vi "Parse string.vi"(11 "Address":string) -> (0 "Len":u8, 1 "StartAddress":u32, 2 "DataBlock":u16, 3 "Memory Area":T1=enum."DB Area")   [LabVIEW 2025, in "SIMATIC_S7.lvclass"]
uses:
  SIMATIC_S7.lvclass
  <vilib>/Hampel Software Engineering/S7NetCom/Source/Controls/S7_Memory_Area.ctl
  <vilib>/regexp/Match Regular Expression.xnode
  <vilib>/Hampel Software Engineering/S7NetCom/Source/S7NetCom.lvclass
panel:
  # "DB6010.40[28]"
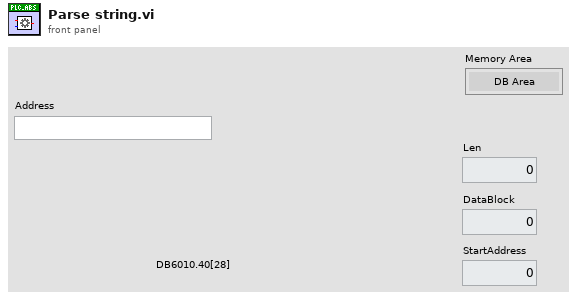
[diagram p1: front panel]
types:
  T1 = typedef "S7NetCom.lvlib/S7NetCom.lvclass/S7_Memory_Area.ctl" = enum8{"P Area", "I Area", "O Area", "M Area", "DB Area", "Counter", "Timer"}
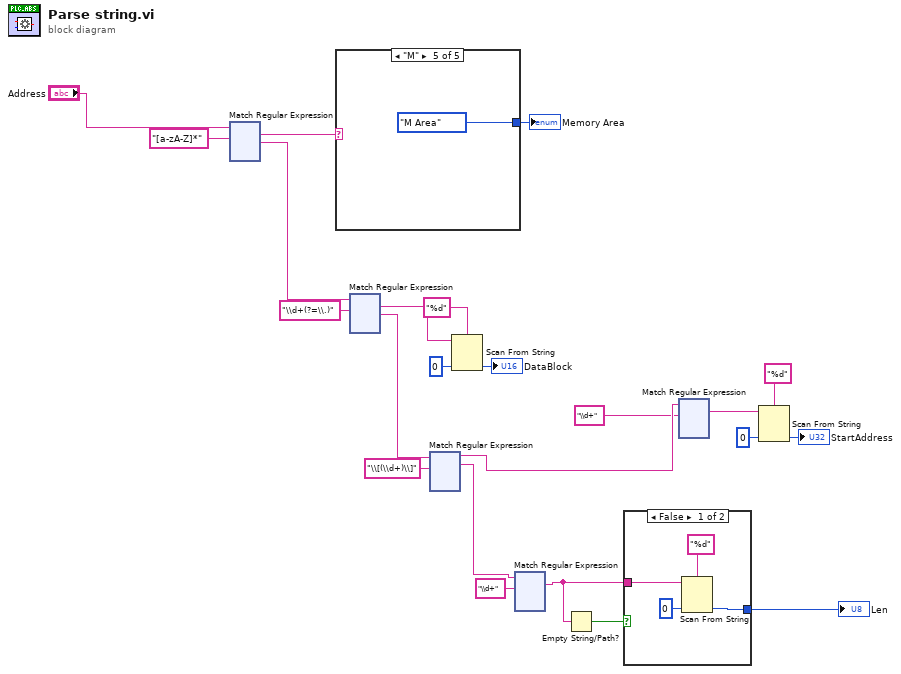
[diagram p0: block diagram]
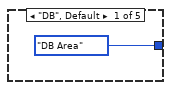
[diagram p3: hidden frame]
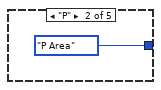
[diagram p4: hidden frame]
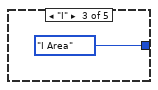
[diagram p5: hidden frame]
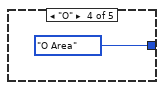
[diagram p6: hidden frame]
diagram:
  n1 = xnode "Match Regular Expression"("input string"="Address", "regular expression"="[a-zA-Z]*") -> ("whole match"=w21:string, "after match"=w19:string)  [unwired: 4 in, 3 out]
  n2 = case shown="\"M\"" w21 {
    tunnel: [S7_Memory_Area."DB Area" ("Memory Area") S7_Memory_Area."P Area" ("Memory Area") S7_Memory_Area."I Area" ("Memory Area") S7_Memory_Area."O Area" ("Memory Area") S7_Memory_Area."M Area" ("Memory Area")] -> w20
    frame "DB", Default {
    }
    frame "P" {
    }
    frame "I" {
    }
    frame "O" {
    }
    frame "M" {
    }
  }
  "Memory Area" <- w20
  n3 = xnode "Match Regular Expression"("input string"=w19, "regular expression"="\\d+(?=\\.)") -> ("whole match"=w17:string, "after match"=w14:string)  [unwired: 4 in, 3 out]
  n4 = xnode "Match Regular Expression"("input string"=w14, "regular expression"="\\[(\\d+)\\]") -> ("before match"=w12:string, "whole match"=w6:string)  [unwired: 4 in, 3 out]
  n5 = Scan From String(format string="%d", input string=w17, default 1=u16 0 ("default value 14")) -> (output 1=→"DataBlock":u16)  [unwired: 2 in, 3 out]
  n6 = xnode "Match Regular Expression"("input string"=w6, "regular expression"="\\d+") -> ("whole match"=w4:string)  [unwired: 4 in, 4 out]
  n7 = Empty String/Path?(string/path=w4) -> (empty?=w3:bool)
  n8 = case shown="False" w3 {
    tunnel: [w31 _] -> w5
    tunnel: w4 -> [w30 _]
    frame False {
      n9 = Scan From String(format string="%d", input string=w30, default 1=u8 0 ("default value 14")) -> (output 1=w31:u8)  [unwired: 2 in, 3 out]
    }
    frame True {
    }
  }
  "Len" <- w5
  n10 = xnode "Match Regular Expression"("input string"=w12, "regular expression"="\\d+") -> ("whole match"=w10:string)  [unwired: 4 in, 4 out]
  n11 = Scan From String(format string="%d", input string=w10, default 1=u32 0 ("default value 14")) -> (output 1=→"StartAddress":u32)  [unwired: 2 in, 3 out]
